vi "MT Map ASK Symbols to Bits.vi"(0 "symbols":cdb[](array[numeric]) format="%.2f", 5 "symbol map":cdb[](array[numeric]) format="%.3f", 11 "error in (no error)":errorcluster) -> (4 "output bit stream":i8[](array[numeric]), 15 "error out":errorcluster)   [LabVIEW 2020, in "niDMT.lvlib"]
doc: "This polymorphic instance maps complex-valued ASK symbols to an <B>output bit stream</B> based on a user-specified symbol map."
uses:
  <vilib>/addons/Modulation/niDMT.lvlib
  <vilib>/addons/Modulation/niAMT.lvlib
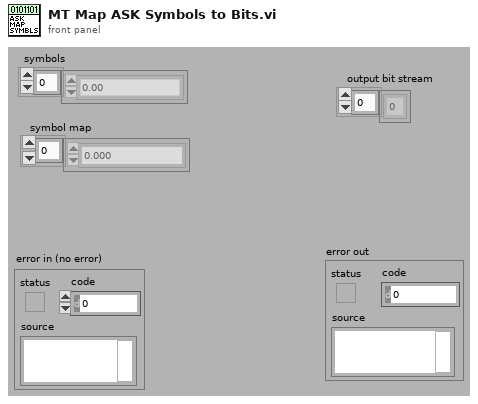
[diagram p1: front panel]
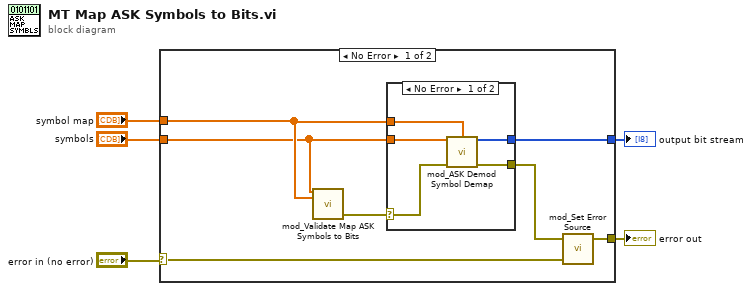
[diagram p0: block diagram]
diagram:
  n1 = case shown="No Error" "error in (no error)" {
    selector: "error in (no error)" -> [w10 w19]
    tunnel: "symbols" -> [w6 _]
    tunnel: [w9 w19] -> w3
    tunnel: [w12 _] -> w2
    tunnel: "symbol map" -> [w7 _]
    frame No Error {
      n2 = call <vilib>:"mod_Validate Map ASK Symbols to Bits.vi"("symbols"=w6, "symbol map"=w7) -> ("error out"=w11:errorcluster)  [unwired: 13 out]
      n3 = case shown="No Error" w11 {
        selector: w11 -> [w14 w18]
        tunnel: w6 -> [w17 _]
        tunnel: [w16 w18] -> w8
        tunnel: [w15 _] -> w12
        tunnel: w7 -> [w13 _]
        frame No Error {
          n4 = call <vilib>:"mod_ASK Demod Symbol Demap.vi"("Symbols In"=w17, "Symbol Map"=w13, "error in (no error)"=w14) -> ("Bits Out"=w15:i8[], "error out"=w16:errorcluster)  [unwired: 11 out]
        }
        frame Error {
        }
      }
      n5 = call <vilib>:"mod_Set Error Source.vi"("initial error in (no error)"=w10, "final error in (no error)"=w8) -> ("error out"=w9:errorcluster)  [unwired: 3 out]
    }
    frame Error {
    }
  }
  "error out" <- w3
  "output bit stream" <- w2
